vi "Monitor Select Demo.vi"() -> ()   [LabVIEW 2013]
panel:
  out "time":string
  in  "Quit":bool
  in  "Monitor Select":bool
  # "VI Properties MUST be set:"
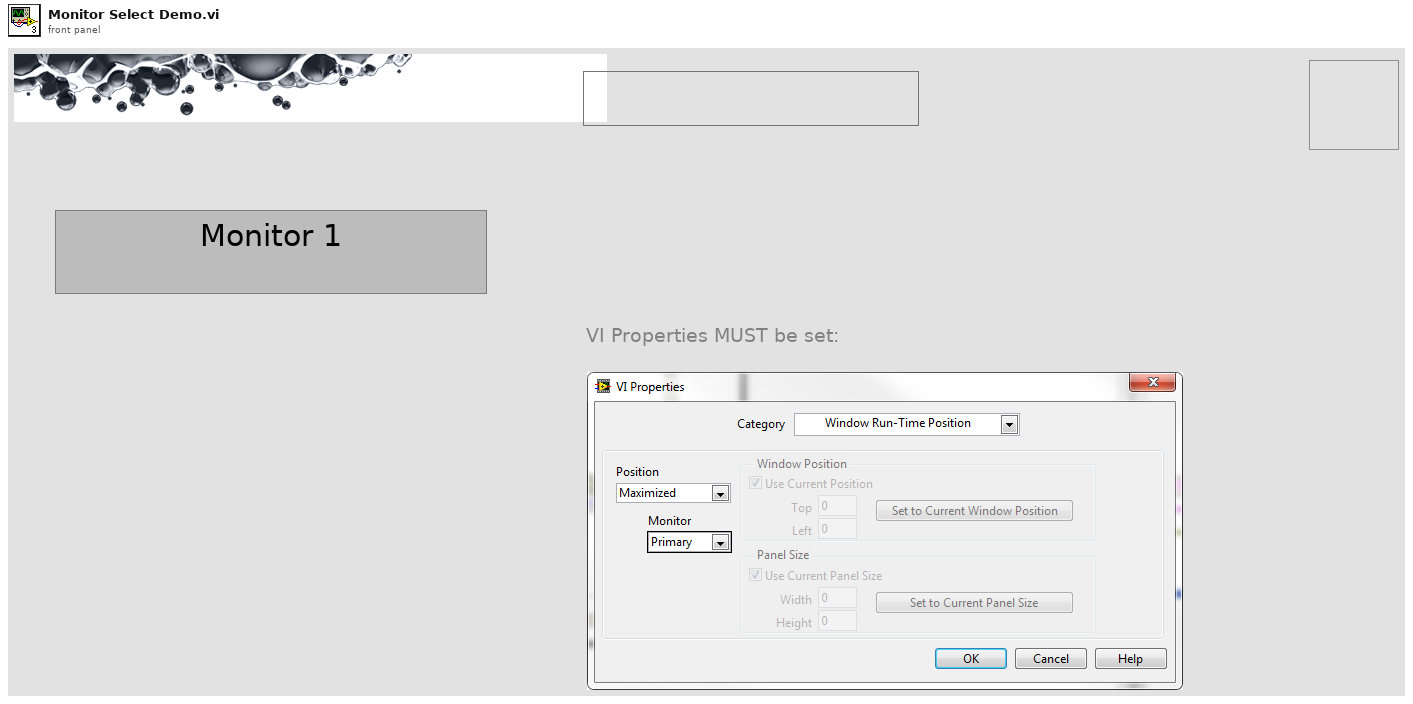
[diagram p1: front panel]
types:
  T1 = enum32{"Invalid", "Standard", "Closed", "Hidden", "Minimized", "Maximized"}
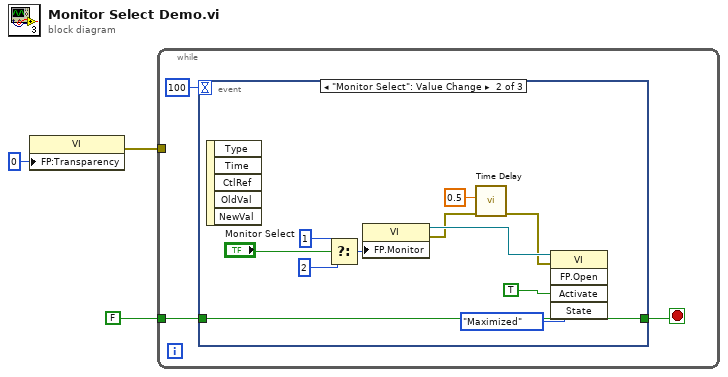
[diagram p0: block diagram]
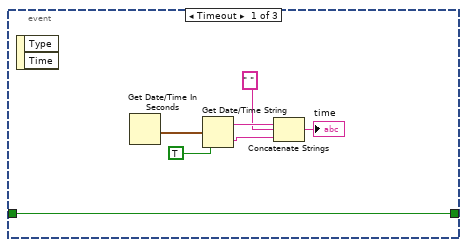
[diagram p2: hidden frame]
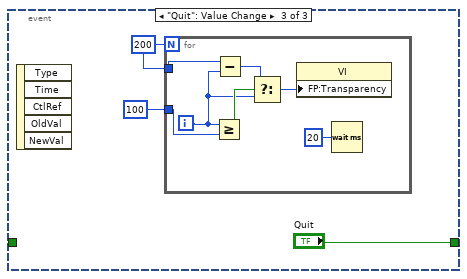
[diagram p3: hidden frame]
diagram:
  n1 = property class="VI"("FP:Transparency"=u8 0 ("Front Panel Window:Transparency")) -> (error out=w1:errorcluster)  [unwired: 2 in, 1 out]
  n2 = while {
    tunnel: FALSE -> [w5]
    tunnel: w1 -> [_]
    stop <- w4 stop-if-true
    n3 = event shown="[1] \"Monitor Select\": Value Change" {
      selector: _ -> [_ _ _]
      dyn-events: _ -> [_ _ _]
      timeout: 100 -> [_ _ _]
      tunnel: [w13 w20 "Quit"] -> w4
      tunnel: w5 -> [w13 w20 _]
      event Timeout {
        n4 = event-data() -> ()  [unwired: 1 in, 2 out]
        n5 = Get Date/Time In Seconds() -> (seconds since 1Jan1904=w7:timestamp)
        n6 = Get Date/Time String(seconds (now)=w7, want seconds? (F)=TRUE) -> (date string=w12:string, time string=w11:string)  [unwired: 1 in]
        n7 = Concatenate Strings(w12, " ", w11) -> (→"time":string)
      }
      event "Monitor Select": Value Change {
        n8 = event-data() -> ()  [unwired: 1 in, 5 out]
        n9 = Select(t=u16 1 ("Front Panel Window:Monitor"), s="Monitor Select", f=u16 2 ("Front Panel Window:Monitor")) -> (s? t:f=w24:u16)
        n10 = property class="VI"("FP.Monitor"=w24) -> (reference out=w19:refnum<vi>, error out=w15:errorcluster)  [unwired: 2 in]
        n11 = call "Time Delay"("error in (no error)"=w15, "Delay Time (s)"=0.5) -> ("error out"=w14:errorcluster)  [unwired: 9 in]
        n12 = invoke class="VI" method="FP.Open"(reference=w19, error in=w14, "Activate"=TRUE, "State"=T1."Maximized") -> ()  [unwired: 1 in, 5 out]
      }
      event "Quit": Value Change {
        w26 = 200
        n13 = event-data() -> ()  [unwired: 1 in, 5 out]
        n14 = for {
          N: w26 -> [_]
          tunnel: w26 -> [w30]
          tunnel: 100 -> [w33]
          i -> [w29]
          n15 = Greater Or Equal?(x=w29, y=w33) -> (x >= y?=w32:bool)
          n16 = Subtract(x=w30, y=w29) -> (x-y=w28:i32)
          n17 = Select(t=w28, s=w32, f=w29) -> (s? t:f=w31:i32)
          n18 = property class="VI"("FP:Transparency"=w31) -> ()  [unwired: 2 in, 2 out]
          n19 = Wait (ms)(milliseconds to wait=u32 20) -> ()  [unwired: 1 out]
        }
      }
    }
  }
